vi "BPM to LEDs.vi"(11 "LEDs":T1) -> ()   [LabVIEW 2015]
uses:
  <vilib>/rvi/eio/common/nirviEmuTemplateMethod_errors.vi
  <vilib>/eio/EIONode/EIONode.xnode
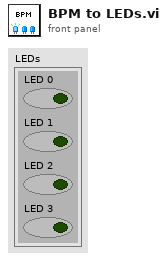
[diagram p1: front panel]
types:
  T1 = cluster{"LED 0":bool, "LED 1":bool, "LED 2":bool, "LED 3":bool}
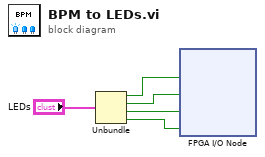
[diagram p0: block diagram]
diagram:
  n1 = Unbundle("LEDs") -> ("LED 0"=w2:bool, "LED 1"=w3:bool, "LED 2"=w4:bool, "LED 3"=w5:bool)
  n2 = xnode "FPGA I/O Node"("LED0"=w2, "LED1"=w3, "LED2"=w4, "LED3"=w5) -> ()  [unwired: 4 in, 4 out]
